vi "ZNB initialization.vi"(8 "error in (no error)":errorcluster, 9 "Output port":i32, 10 "Input port":i32, 11 "VISA resource name":refnum<visa-resource-name>) -> (0 "error out":errorcluster, 3 "VISA resource name out":refnum<visa-resource-name>)   [LabVIEW 2015]
uses:
  <instrlib>/Rohde&Schwarz Vector Network Analyzer/Rohde&Schwarz Vector Network Analyzer.lvlib
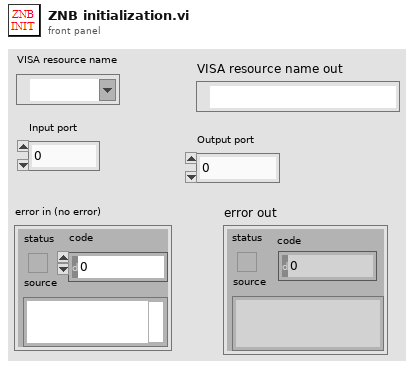
[diagram p1: front panel]
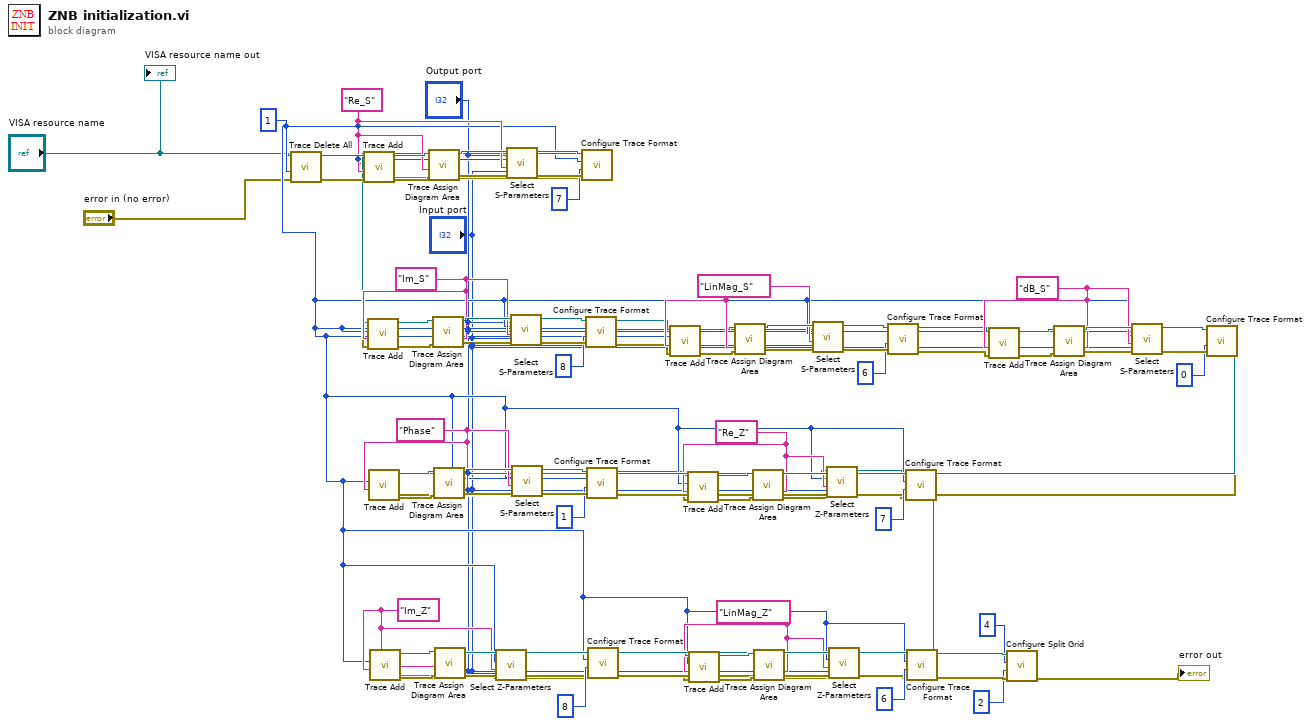
[diagram p0: block diagram]
diagram:
  w21 = "LinMag_Z"
  w22 = "Im_Z"
  w25 = "Re_Z"
  w49 = "Phase"
  w57 = "dB_S"
  w65 = "LinMag_S"
  w75 = "Im_S"
  w76 = "Re_S"
  w20 = 1
  n1 = call <instrlib>:"Trace Delete All.vi"("error in (no error)"="error in (no error)", "Channel (1)"=w20, "VISA resource name"="VISA resource name") -> ("error out"=w89:errorcluster, "VISA resource name out"=w90:refnum<visa-resource-name>)  [unwired: 7 in]
  n2 = call <instrlib>:"Trace Add.vi"("error in (no error)"=w89, "Trace Name (\"Trc1\")"=w76, "Channel (1)"=w20, "VISA resource name"=w90) -> ("error out"=w78:errorcluster, "VISA resource name out"=w77:refnum<visa-resource-name>)  [unwired: 6 in]
  n3 = call <instrlib>:"Trace Assign Diagram Area.vi"("error in (no error)"=w78, "Trace Name (\"Ch1Trc1\")"=w76, "VISA resource name"=w77) -> ("error out"=w87:errorcluster, "VISA resource name out"=w88:refnum<visa-resource-name>)  [unwired: 7 in]
  n4 = call <instrlib>:"Select S-Parameters.vi"("In Port (1)"="Input port", "Out Port (1)"="Output port", "error in (no error)"=w87, "Trace Name (\"Trc1\")"=w76, "Channel (1)"=w20, "VISA resource name"=w88) -> ("error out"=w85:errorcluster, "VISA resource name out"=w86:refnum<visa-resource-name>)  [unwired: 4 in]
  n5 = call <instrlib>:"Configure Trace Format.vi"("error in (no error)"=w85, "Format (dB Mag)"=7, "Channel (1)"=w20, "VISA resource name"=w86) -> ("error out"=w73:errorcluster, "VISA resource name out"=w74:refnum<visa-resource-name>)  [unwired: 6 in]
  n6 = call <instrlib>:"Trace Add.vi"("error in (no error)"=w73, "Trace Name (\"Trc1\")"=w75, "Channel (1)"=w20, "VISA resource name"=w74) -> ("error out"=w71:errorcluster, "VISA resource name out"=w72:refnum<visa-resource-name>)  [unwired: 6 in]
  n7 = call <instrlib>:"Trace Assign Diagram Area.vi"("error in (no error)"=w71, "Trace Name (\"Ch1Trc1\")"=w75, "VISA resource name"=w72) -> ("error out"=w82:errorcluster, "VISA resource name out"=w83:refnum<visa-resource-name>)  [unwired: 7 in]
  n8 = call <instrlib>:"Select S-Parameters.vi"("In Port (1)"="Input port", "Out Port (1)"="Output port", "error in (no error)"=w82, "Trace Name (\"Trc1\")"=w75, "Channel (1)"=w20, "VISA resource name"=w83) -> ("error out"=w80:errorcluster, "VISA resource name out"=w81:refnum<visa-resource-name>)  [unwired: 4 in]
  n9 = call <instrlib>:"Configure Trace Format.vi"("error in (no error)"=w80, "Format (dB Mag)"=8, "Channel (1)"=w20, "VISA resource name"=w81) -> ("error out"=w36:errorcluster, "VISA resource name out"=w37:refnum<visa-resource-name>)  [unwired: 6 in]
  n10 = call <instrlib>:"Trace Add.vi"("error in (no error)"=w36, "Trace Name (\"Trc1\")"=w65, "Channel (1)"=w20, "VISA resource name"=w37) -> ("error out"=w63:errorcluster, "VISA resource name out"=w64:refnum<visa-resource-name>)  [unwired: 6 in]
  n11 = call <instrlib>:"Trace Assign Diagram Area.vi"("error in (no error)"=w63, "Trace Name (\"Ch1Trc1\")"=w65, "VISA resource name"=w64) -> ("error out"=w69:errorcluster, "VISA resource name out"=w70:refnum<visa-resource-name>)  [unwired: 7 in]
  n12 = call <instrlib>:"Select S-Parameters.vi"("In Port (1)"="Input port", "Out Port (1)"="Output port", "error in (no error)"=w69, "Trace Name (\"Trc1\")"=w65, "Channel (1)"=w20, "VISA resource name"=w70) -> ("error out"=w67:errorcluster, "VISA resource name out"=w68:refnum<visa-resource-name>)  [unwired: 4 in]
  n13 = call <instrlib>:"Configure Trace Format.vi"("error in (no error)"=w67, "Format (dB Mag)"=6, "VISA resource name"=w68) -> ("error out"=w34:errorcluster, "VISA resource name out"=w35:refnum<visa-resource-name>)  [unwired: 7 in]
  n14 = call <instrlib>:"Trace Add.vi"("error in (no error)"=w34, "Trace Name (\"Trc1\")"=w57, "VISA resource name"=w35) -> ("error out"=w55:errorcluster, "VISA resource name out"=w56:refnum<visa-resource-name>)  [unwired: 7 in]
  n15 = call <instrlib>:"Trace Assign Diagram Area.vi"("error in (no error)"=w55, "Trace Name (\"Ch1Trc1\")"=w57, "VISA resource name"=w56) -> ("error out"=w61:errorcluster, "VISA resource name out"=w62:refnum<visa-resource-name>)  [unwired: 7 in]
  n16 = call <instrlib>:"Select S-Parameters.vi"("In Port (1)"="Input port", "Out Port (1)"="Output port", "error in (no error)"=w61, "Trace Name (\"Trc1\")"=w57, "Channel (1)"=w20, "VISA resource name"=w62) -> ("error out"=w59:errorcluster, "VISA resource name out"=w60:refnum<visa-resource-name>)  [unwired: 4 in]
  n17 = call <instrlib>:"Configure Trace Format.vi"("error in (no error)"=w59, "Format (dB Mag)"=0, "VISA resource name"=w60) -> ("error out"=w32:errorcluster, "VISA resource name out"=w33:refnum<visa-resource-name>)  [unwired: 7 in]
  n18 = call <instrlib>:"Trace Add.vi"("error in (no error)"=w32, "Trace Name (\"Trc1\")"=w49, "Channel (1)"=w20, "VISA resource name"=w33) -> ("error out"=w47:errorcluster, "VISA resource name out"=w48:refnum<visa-resource-name>)  [unwired: 6 in]
  n19 = call <instrlib>:"Trace Assign Diagram Area.vi"("error in (no error)"=w47, "Trace Name (\"Ch1Trc1\")"=w49, "VISA resource name"=w48) -> ("error out"=w53:errorcluster, "VISA resource name out"=w54:refnum<visa-resource-name>)  [unwired: 7 in]
  n20 = call <instrlib>:"Select S-Parameters.vi"("In Port (1)"="Input port", "Out Port (1)"="Output port", "error in (no error)"=w53, "Trace Name (\"Trc1\")"=w49, "Channel (1)"=w20, "VISA resource name"=w54) -> ("error out"=w51:errorcluster, "VISA resource name out"=w52:refnum<visa-resource-name>)  [unwired: 4 in]
  n21 = call <instrlib>:"Configure Trace Format.vi"("error in (no error)"=w51, "Format (dB Mag)"=1, "Channel (1)"=w20, "VISA resource name"=w52) -> ("error out"=w16:errorcluster, "VISA resource name out"=w17:refnum<visa-resource-name>)  [unwired: 6 in]
  n22 = call <instrlib>:"Trace Add.vi"("error in (no error)"=w16, "Trace Name (\"Trc1\")"=w25, "Channel (1)"=w20, "VISA resource name"=w17) -> ("error out"=w44:errorcluster, "VISA resource name out"=w45:refnum<visa-resource-name>)  [unwired: 6 in]
  n23 = call <instrlib>:"Trace Assign Diagram Area.vi"("error in (no error)"=w44, "Trace Name (\"Ch1Trc1\")"=w25, "VISA resource name"=w45) -> ("error out"=w14:errorcluster, "VISA resource name out"=w15:refnum<visa-resource-name>)  [unwired: 7 in]
  n24 = call <instrlib>:"Select Z-Parameters.vi"("In Port (1)"="Input port", "Out Port (1)"="Output port", "error in (no error)"=w14, "Trace Name (\"Trc1\")"=w25, "Channel (1)"=w20, "VISA resource name"=w15) -> ("error out"=w23:errorcluster, "VISA resource name out"=w24:refnum<visa-resource-name>)  [unwired: 4 in]
  n25 = call <instrlib>:"Configure Trace Format.vi"("error in (no error)"=w23, "Format (dB Mag)"=7, "Channel (1)"=w20, "VISA resource name"=w24) -> ("error out"=w30:errorcluster, "VISA resource name out"=w31:refnum<visa-resource-name>)  [unwired: 6 in]
  n26 = call <instrlib>:"Trace Add.vi"("error in (no error)"=w30, "Trace Name (\"Trc1\")"=w22, "Channel (1)"=w20, "VISA resource name"=w31) -> ("error out"=w41:errorcluster, "VISA resource name out"=w42:refnum<visa-resource-name>)  [unwired: 6 in]
  n27 = call <instrlib>:"Trace Assign Diagram Area.vi"("error in (no error)"=w41, "Trace Name (\"Ch1Trc1\")"=w22, "VISA resource name"=w42) -> ("error out"=w12:errorcluster, "VISA resource name out"=w13:refnum<visa-resource-name>)  [unwired: 7 in]
  n28 = call <instrlib>:"Select Z-Parameters.vi"("In Port (1)"="Input port", "Out Port (1)"="Output port", "error in (no error)"=w12, "Trace Name (\"Trc1\")"=w22, "Channel (1)"=w20, "VISA resource name"=w13) -> ("error out"=w28:errorcluster, "VISA resource name out"=w29:refnum<visa-resource-name>)  [unwired: 4 in]
  n29 = call <instrlib>:"Configure Trace Format.vi"("error in (no error)"=w28, "Format (dB Mag)"=8, "Channel (1)"=w20, "VISA resource name"=w29) -> ("error out"=w26:errorcluster, "VISA resource name out"=w27:refnum<visa-resource-name>)  [unwired: 6 in]
  n30 = call <instrlib>:"Trace Add.vi"("error in (no error)"=w26, "Trace Name (\"Trc1\")"=w21, "Channel (1)"=w20, "VISA resource name"=w27) -> ("error out"=w38:errorcluster, "VISA resource name out"=w39:refnum<visa-resource-name>)  [unwired: 6 in]
  n31 = call <instrlib>:"Trace Assign Diagram Area.vi"("error in (no error)"=w38, "Trace Name (\"Ch1Trc1\")"=w21, "VISA resource name"=w39) -> ("error out"=w10:errorcluster, "VISA resource name out"=w11:refnum<visa-resource-name>)  [unwired: 7 in]
  n32 = call <instrlib>:"Select Z-Parameters.vi"("In Port (1)"="Input port", "Out Port (1)"="Output port", "error in (no error)"=w10, "Trace Name (\"Trc1\")"=w21, "Channel (1)"=w20, "VISA resource name"=w11) -> ("error out"=w8:errorcluster, "VISA resource name out"=w9:refnum<visa-resource-name>)  [unwired: 4 in]
  n33 = call <instrlib>:"Configure Trace Format.vi"("error in (no error)"=w8, "Format (dB Mag)"=6, "Channel (1)"=w20, "VISA resource name"=w9) -> ("error out"=w6:errorcluster, "VISA resource name out"=w7:refnum<visa-resource-name>)  [unwired: 6 in]
  n34 = call <instrlib>:"Configure Split Grid.vi"("error in (no error)"=w6, "Columns (1)"=2, "Rows (1)"=4, "VISA resource name"=w7) -> ("error out"=→"error out":errorcluster)  [unwired: 6 in, 1 out]
  "VISA resource name out" <- "VISA resource name"
